vi "JoystickPercentPressed.Hashtag.vi"(1 "X input":dbl, 2 "Y input":dbl) -> (0 "Percentage":dbl)   [LabVIEW 2014]
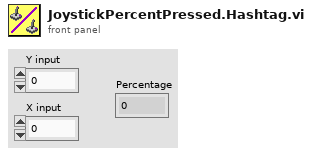
[diagram p1: front panel]
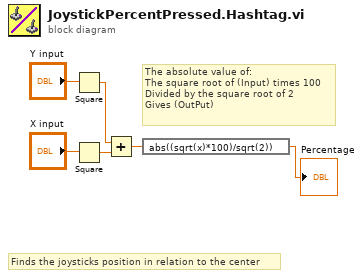
[diagram p0: block diagram]
diagram:
  # "Finds the joysticks position in relation to the center"
  # "The absolute value of:\nThe square root of (Input) times 100\nDivided by the square root of 2\nGives (OutPut)"
  n1 = Square(x="Y input") -> (x^2=w5:dbl)
  n2 = Square(x="X input") -> (x^2=w6:dbl)
  n3 = Add(x=w5, y=w6) -> (x+y=w4:dbl)
  n4 = expression code="abs((sqrt(x)*100)/sqrt(2))"(w4) -> (→"Percentage":dbl)
